vi "Ref Equals.vi"(8 "error in (no error)":errorcluster, 10 "BetterHandle in":refnum<class "BetterHandle.lvclass">, 11 "BetterDropOp in":refnum<class "BetterDropOp.lvclass">) -> (0 "error out":errorcluster, 1 "DragStart Indices":i32[](array[numeric]), 2 "Ref is same?":bool, 3 "BetterDropOp out":refnum<class "BetterDropOp.lvclass">)   [LabVIEW 2020, in "BetterDragAndDrop.lvlib" / "BetterDropOp.lvclass"]
uses:
  BetterDropOp.lvclass
  BetterHandle/BetterHandle.lvclass
  BetterDropOp.lvclass/BetterDropOp.ctl
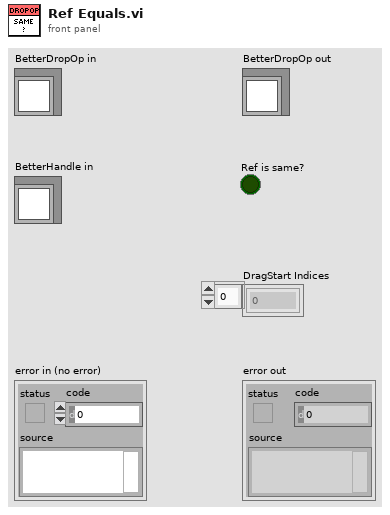
[diagram p1: front panel]
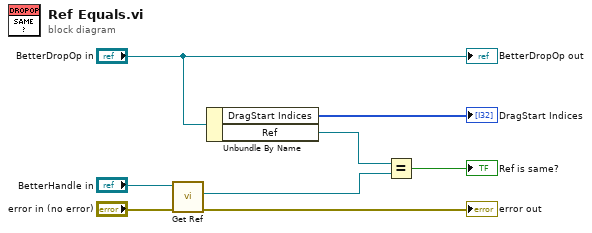
[diagram p0: block diagram]
diagram:
  n1 = call-dynamic "Get Ref.vi"("error in (no error)"="error in (no error)", "BetterHandle in"="BetterHandle in") -> ("error out"=→"error out":errorcluster, "Tree/LB/MCL ref"=w1:refnum<vi>)  [unwired: 7 in, 1 out]
  n2 = Unbundle By Name("BetterDropOp in") -> ("DragStart Indices"=→"DragStart Indices":i32[], "Ref"=w8:refnum<vi>)
  n3 = Equal?(x=w8, y=w1) -> (x = y?=→"Ref is same?":bool)
  "BetterDropOp out" <- "BetterDropOp in"
